vi "Specify_path_DCDC_Dura.vi"(5 "Path_Enum":enum16{"Find_Path", "Get_Path"}(ring)=enum."Get_Path", 11 "error in (no error)":errorcluster) -> (2 "Application Directory":path, 3 "stripped path":path, 4 "Configurations":path, 6 "DATA":path, 10 "Settings":path, 14 "path":path, 15 "error out":errorcluster)   [LabVIEW 2025]
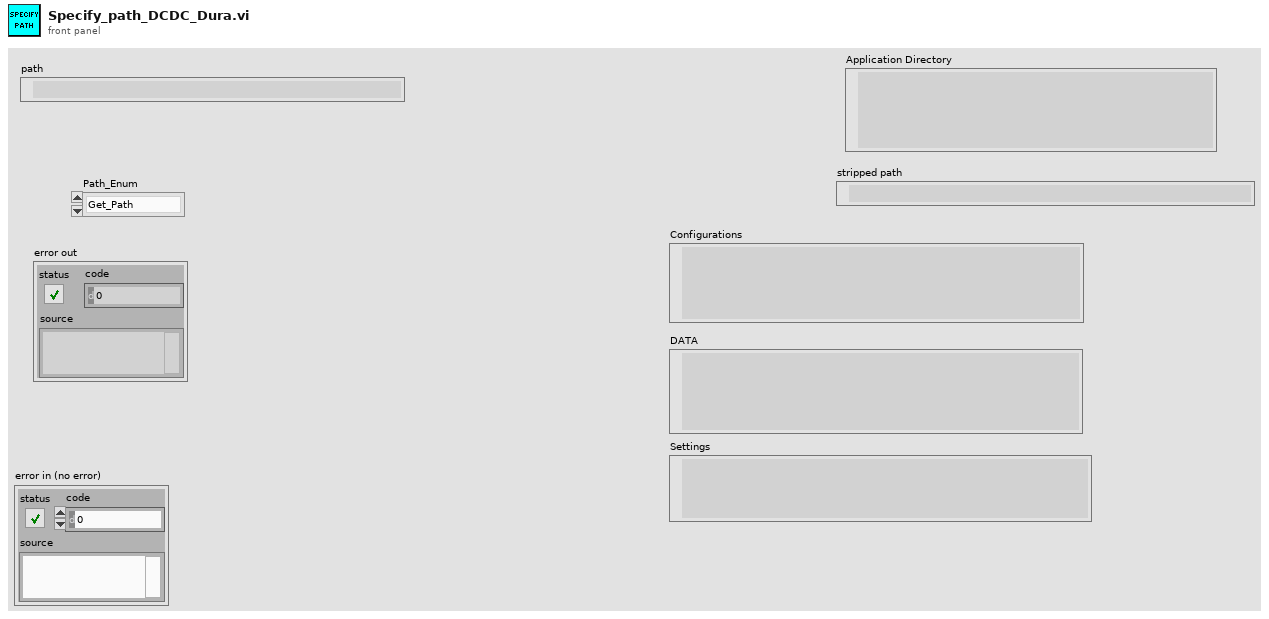
[diagram p1: front panel]
types:
  T1 = enum32{"invalid app kind", "Development System", "Run Time System", "Student Edition", "Embedded LabVIEW", "Evaluation", "Custom"}
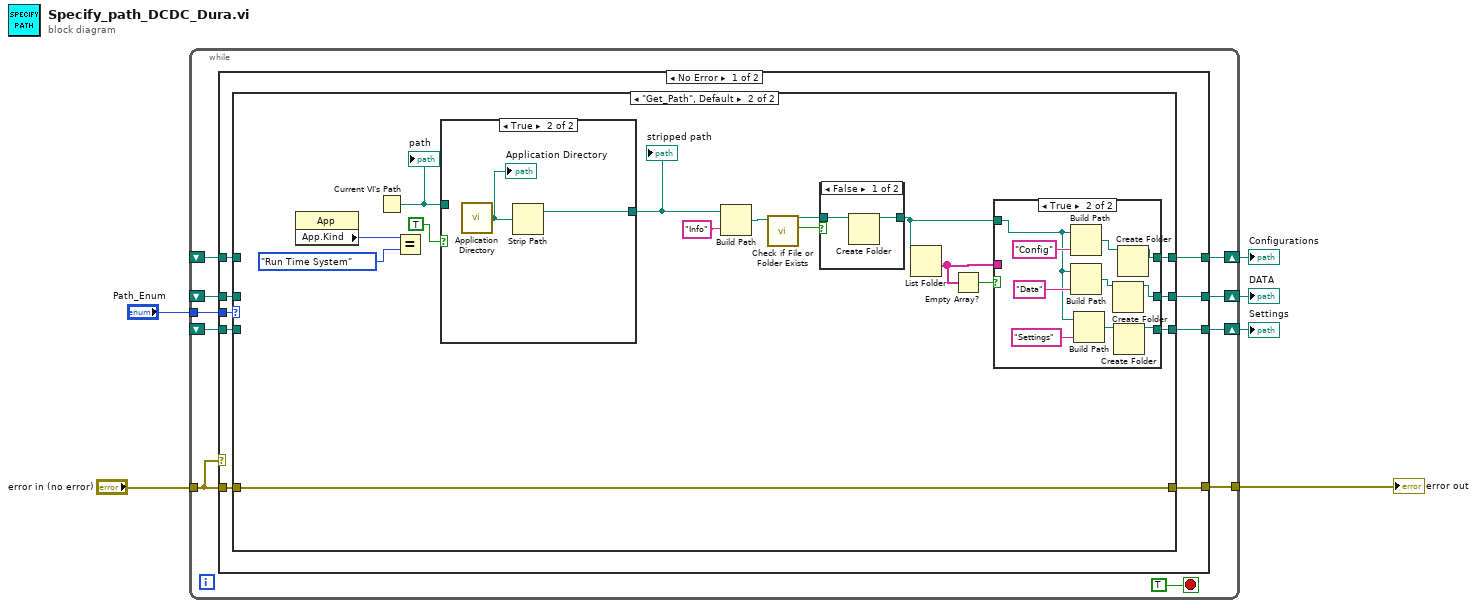
[diagram p0: block diagram]
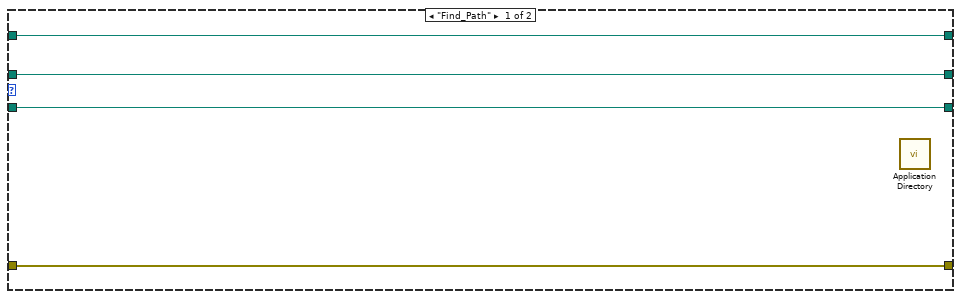
[diagram p2: hidden frame]
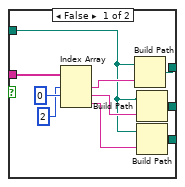
[diagram p3: hidden frame]
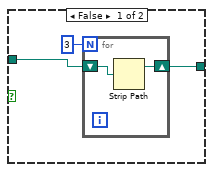
[diagram p5: hidden frame]
diagram:
  n1 = while {
    tunnel: "error in (no error)" -> [w15]
    tunnel: [w14] -> w5
    tunnel: "Path_Enum" -> [w13]
    shift-right: [w12] -> w3
    shift-left: _ -> [w10]
    shift-right: [w11] -> w2
    shift-left: _ -> [w9]
    shift-right: [w8] -> w1
    shift-left: _ -> [w7]
    stop <- TRUE stop-if-true
    n2 = case shown="No Error" w15 {
      tunnel: w15 -> [w25 w76]
      tunnel: [w24 w76] -> w14
      tunnel: w13 -> [w23 _]
      tunnel: [w22 _] -> w12
      tunnel: [w21 _] -> w11
      tunnel: w10 -> [w20 _]
      tunnel: w9 -> [w19 _]
      tunnel: [w18 _] -> w8
      tunnel: w7 -> [w17 _]
      frame No Error {
        n3 = case shown="\"Get_Path\", Default" w23 {
          tunnel: w25 -> [w29 w45]
          tunnel: [w29 w45] -> w24
          tunnel: [w28 w40] -> w22
          tunnel: [w27 w39] -> w21
          tunnel: w20 -> [w28 _]
          tunnel: w19 -> [w27 _]
          tunnel: [w26 w38] -> w18
          tunnel: w17 -> [w26 _]
          frame "Find_Path" {
            n4 = call <vilib>:"Application Directory.vi"() -> ()  [unwired: 1 out]
          }
          frame "Get_Path", Default {
            n5 = property class="App"() -> ("App.Kind"=w44:T1)  [unwired: 2 in, 2 out]
            n6 = Current VI's Path() -> (path=w42:path)
            "path" <- w42
            n7 = Equal?(x=w44, y=T1."Run Time System" ("Application:Kind")) -> ()  [unwired: 1 out]
            n8 = case shown="True" TRUE {
              tunnel: w42 -> [w71 _]
              tunnel: [w69 w75] -> w36
              frame False {
                n9 = for {
                  N: 3 -> [_]
                  shift-right: [w72] -> w69
                  shift-left: w71 -> [w73]
                  n10 = Strip Path(path=w73) -> (stripped path=w72:path)  [unwired: 1 out]
                }
              }
              frame True {
                n11 = call <vilib>:"Application Directory.vi"() -> ("Application Directory"=w74:path)
                "Application Directory" <- w74
                n12 = Strip Path(path=w74) -> (stripped path=w75:path)  [unwired: 1 out]
              }
            }
            "stripped path" <- w36
            n13 = Build Path(base path=w36, name or relative path="Info") -> (appended path=w35:path)
            n14 = call <vilib>:"Check if File or Folder Exists.vi"("path"=w35) -> ("file or folder exists?"=w34:bool, "dup path"=w33:path)  [unwired: 8 in, 1 out]
            n15 = case shown="False" w34 {
              tunnel: w33 -> [w67 w68]
              tunnel: [w66 w68] -> w32
              frame False {
                n16 = Create Folder(path (use dialog)=w67) -> (created path=w66:path)  [unwired: 2 in, 2 out]
              }
              frame True {
              }
            }
            n17 = List Folder(path=w32) -> (folder names=w31:string[])  [unwired: 3 in, 3 out]
            n18 = Empty Array?(array=w31) -> (empty?=w30:bool)
            n19 = case shown="True" w30 {
              tunnel: w31 -> [w55 _]
              tunnel: [w52 w61] -> w40
              tunnel: [w51 w60] -> w39
              tunnel: [w49 w58] -> w38
              tunnel: w32 -> [w46 w57]
              frame False {
                n20 = Index Array(array=w55, index #1=2 ("index"), index #2=0 ("index")) -> (element #1=w54:string, element #2=w53:string, element #3=w50:string)  [unwired: 1 in]
                n21 = Build Path(base path=w46, name or relative path=w54) -> (appended path=w52:path)
                n22 = Build Path(base path=w46, name or relative path=w53) -> (appended path=w51:path)
                n23 = Build Path(base path=w46, name or relative path=w50) -> (appended path=w49:path)
              }
              frame True {
                n24 = Build Path(base path=w57, name or relative path="Config") -> (appended path=w62:path)
                n25 = Build Path(base path=w57, name or relative path="Data") -> (appended path=w59:path)
                n26 = Build Path(base path=w57, name or relative path="Settings") -> (appended path=w56:path)
                n27 = Create Folder(path (use dialog)=w59) -> (created path=w60:path)  [unwired: 2 in, 2 out]
                n28 = Create Folder(path (use dialog)=w56) -> (created path=w58:path)  [unwired: 2 in, 2 out]
                n29 = Create Folder(path (use dialog)=w62) -> (created path=w61:path)  [unwired: 2 in, 2 out]
              }
            }
          }
        }
      }
      frame Error {
      }
    }
  }
  "error out" <- w5
  "Configurations" <- w3
  "DATA" <- w2
  "Settings" <- w1
